vi "GetFieldFromProtobufIndexni_protobuf_types_WaveformAttributeValue_attribute.vi"(1 "protobuf index":i32) -> (0 "oneof field name":string)   [LabVIEW 2021, in "ni.protobuf.types.lvlib" / "ni_protobuf_types_WaveformAttributeValue_attribute.lvclass"]
uses:
  ni_protobuf_types_WaveformAttributeValue_attribute.lvclass
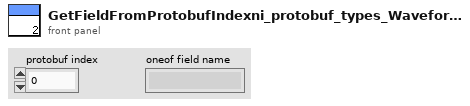
[diagram p1: front panel]
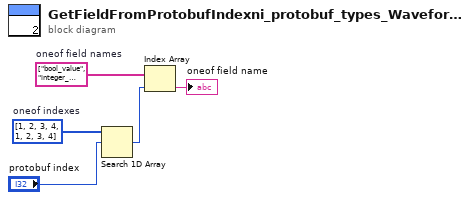
[diagram p0: block diagram]
diagram:
  w5 = string[] ["bool_value", "integer_value", "double_value", "string_value", "bool_value", "integer_value", "double_value", "string_value"]  # oneof field names
  w4 = i32[] [1, 2, 3, 4, 1, 2, 3, 4]  # oneof indexes
  n1 = Search 1D Array(1D array=w4, element="protobuf index") -> (index of element=w2:i32)  [unwired: 1 in]
  n2 = Index Array(array=w5, index=w2) -> (element=→"oneof field name":string)
